vi "From Variant.vi"(0 "Derived in":refnum<class "KDemoDerived.lvclass">, 7 "Variant":variant, 9 "Prefix":string="Derived", 11 "error in (no error)":errorcluster) -> (4 "Derived out":refnum<class "KDemoDerived.lvclass">, 15 "error out":errorcluster)   [LabVIEW 2015, in "KDemoDerived.lvclass"]
uses:
  KDemoDerived.lvclass
  KDemoDerived.lvclass/KDemoDerived.ctl
  KDemoBase Class/KDemoBase.lvclass
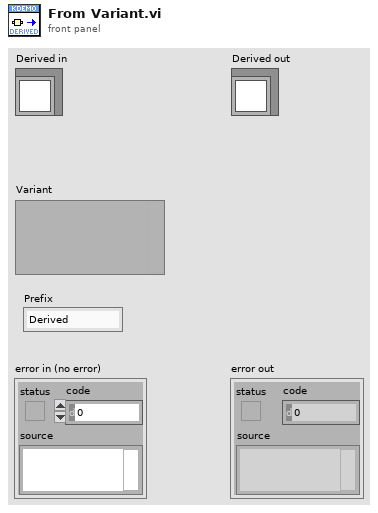
[diagram p1: front panel]
types:
  T1 = typedef "KDemoDerived.lvclass/Serialized.ctl" = cluster{"Integer":i32, "String":string}
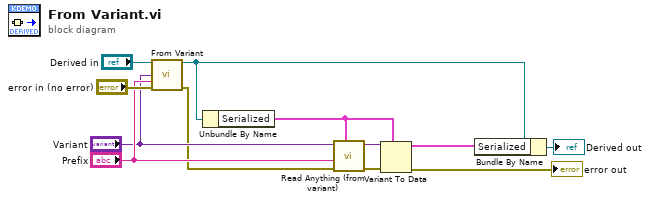
[diagram p0: block diagram]
diagram:
  n1 = call-parent "From Variant.vi"("Derived in"="Derived in", "Variant"="Variant", "Prefix"="Prefix", "error in (no error)"="error in (no error)") -> ("Derived out"=w5:refnum<class "KDemoDerived.lvclass">, "error out"=w7:errorcluster)  [unwired: 10 in]
  n2 = Unbundle By Name(w5) -> ("Serialized"=w3:T1)
  n3 = call "Read Anything (from variant).vi"("Type of Anything"=w3, "Error In"=w7, "Prefix"="Prefix", "Variant Database"="Variant") -> ("Error Out"=w2:errorcluster, "Anything"=w1:variant)  [unwired: 5 in, 1 out]
  n4 = Variant To Data(error in=w2, type=w3, Variant=w1) -> (data=w10:T1, error out=→"error out":errorcluster)
  n5 = Bundle By Name(cluster=w5, "Serialized"=w10) -> (→"Derived out":refnum<class "KDemoDerived.lvclass">)
